vi "Set Rmb User.vi"(8 "error in (no error)":errorcluster, 11 "[User] Cfg File in":refnum<class "[User] Cfg File.lvclass">) -> (0 "error out":errorcluster, 3 "[User] Cfg File out":refnum<class "[User] Cfg File.lvclass">)   [LabVIEW 2020, in "[User] Cfg File.lvclass"]
uses:
  [User] Cfg File.lvclass
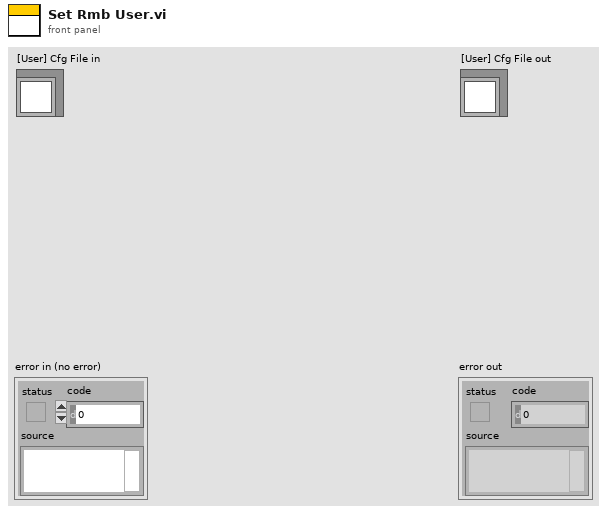
[diagram p1: front panel]
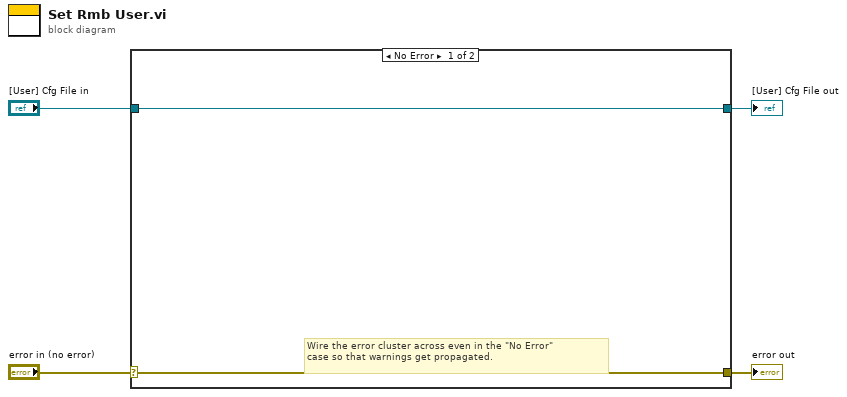
[diagram p0: block diagram]
diagram:
  n1 = case shown="No Error" "error in (no error)" {
    selector: "error in (no error)" -> [w5 w8]
    tunnel: [w5 w8] -> w3
    tunnel: [w6 w7] -> w1
    tunnel: "[User] Cfg File in" -> [w6 w7]
    frame No Error {
      # "Wire the error cluster across even in the \"No Error\"\ncase so that warnings get propagated."
    }
    frame Error {
    }
  }
  "error out" <- w3
  "[User] Cfg File out" <- w1
